vi "Extract 1000330-1 data from report file.vi"() -> ()   [LabVIEW 2013]
panel:
  in  "file (use dialog)":path=path "L:/Synapse/1000330_report_log.txt"
  out "String":string
  out "error out":errorcluster
  in  "error in":errorcluster
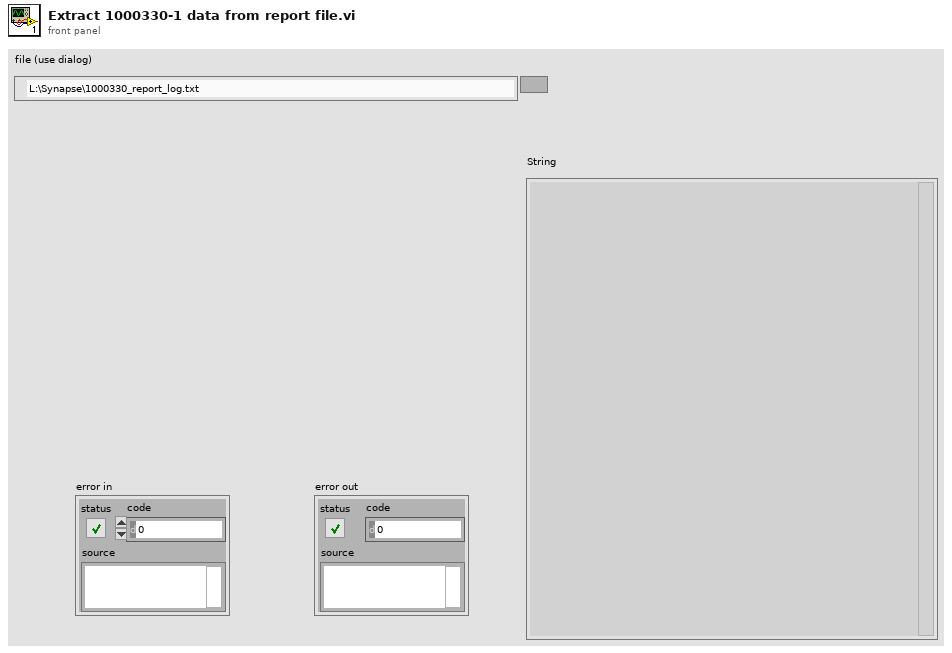
[diagram p1: front panel]
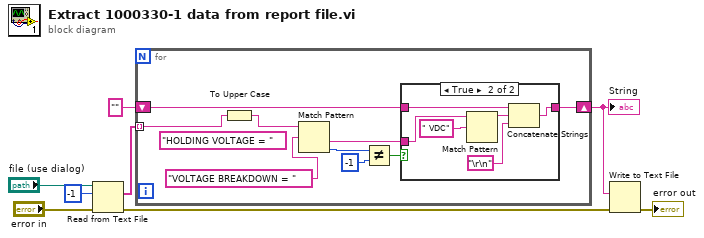
[diagram p0: block diagram]
diagram:
  n1 = Read from Text File(file (use dialog)="file (use dialog)", count=-1, error in="error in") -> (text=w6:string[], error out=w3:errorcluster)  [unwired: 1 in, 2 out]
  n2 = for {
    tunnel: w6 -> [w11] mode=indexing
    shift-right: [w13] -> w4
    shift-left: "" -> [w14]
    (unwired) "HOLDING VOLTAGE = " ("regular expression")
    n3 = To Upper Case(1:w11) -> (0:w10:string)
    n4 = Match Pattern(string=w10, regular expression="VOLTAGE BREAKDOWN = ") -> (after substring=w15:string, offset past match=w16:i32)  [unwired: 1 in, 2 out]
    n5 = Not Equal?(x=w16, y=-1) -> (x != y?=w12:bool)
    n6 = case shown="True" w12 {
      tunnel: w15 -> [_ w23]
      tunnel: w14 -> [w18 w22]
      tunnel: [w18 w20] -> w13
      frame False {
      }
      frame True {
        n7 = Match Pattern(string=w23, regular expression=" VDC") -> (before substring=w21:string)  [unwired: 1 in, 3 out]
        n8 = Concatenate Strings(w22, w21, "\r\n") -> (w20:string)
      }
    }
  }
  "String" <- w4
  n9 = Write to Text File(text=w4, error in=w3) -> (error out=→"error out":errorcluster)  [unwired: 2 in, 2 out]
